vi "load.vi"(8 "error in (no error)":errorcluster, 10 "child node in":refnum<k20>, 11 "TTL_input in":refnum<class "TTL_input.lvclass">) -> (0 "error out":errorcluster, 2 "child node out":refnum<k20>, 3 "TTL_input out":refnum<class "TTL_input.lvclass">)   [LabVIEW 2013, in "TTL_input.lvclass"]
uses:
  TTL_input.lvclass
  TTL_input.lvclass/TTL_input.ctl
  Globals.vi
  <vilib>/xml/Close Reference(Node).vi
  <resource>/objmgr/DOMUserDefRef.rc
  <vilib>/xml/NI_XML.lvlib
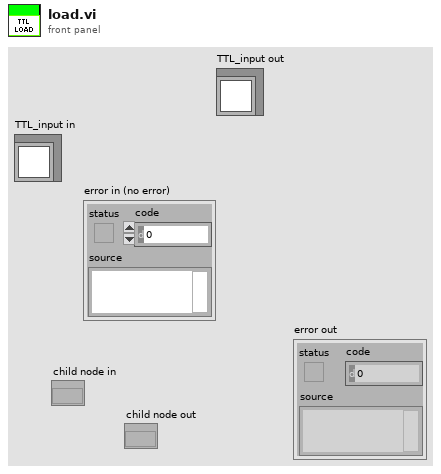
[diagram p1: front panel]
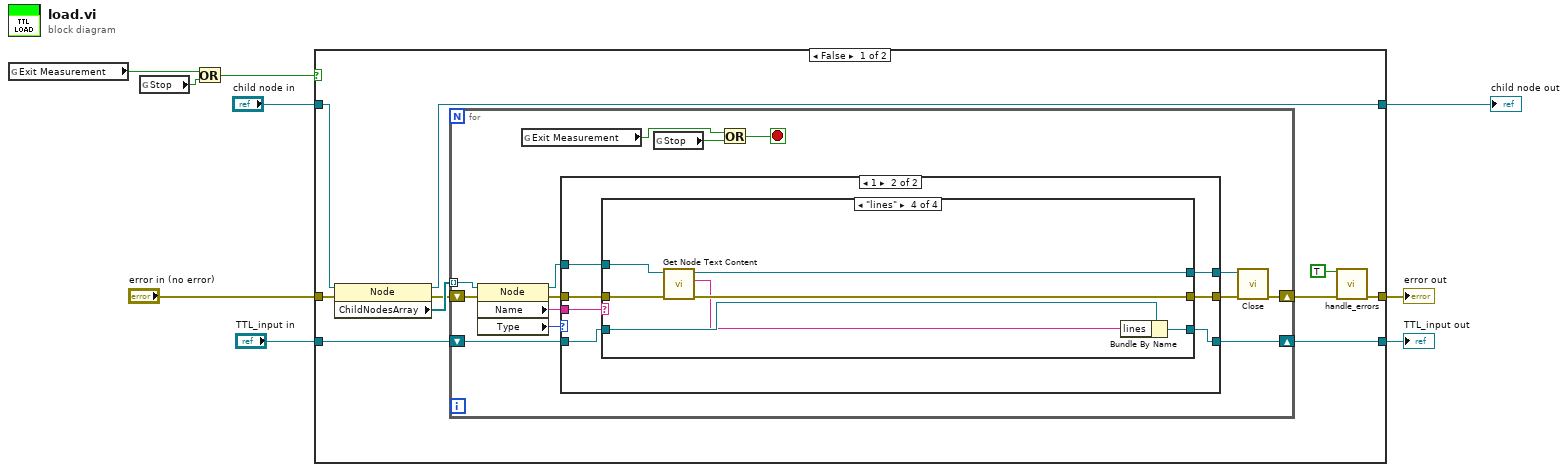
[diagram p0: block diagram]
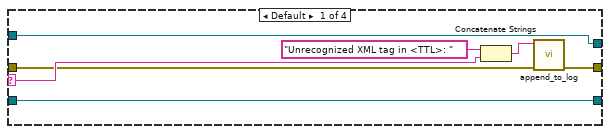
[diagram p3: hidden frame]
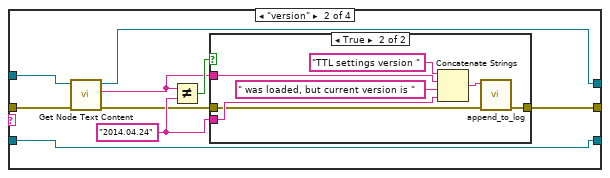
[diagram p4: hidden frame]
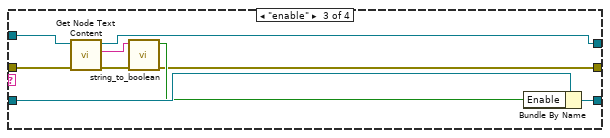
[diagram p6: hidden frame]
diagram:
  n1 = global read "Globals.vi" "Exit Measurement"() -> (w9:bool)
  n2 = global read "Globals.vi" "Stop"() -> (w8:bool)
  n3 = Or(x=w9, y=w8) -> (x .or. y?=w7:bool)
  n4 = case shown="False" w7 {
    tunnel: [w18 w86] -> w3
    tunnel: "error in (no error)" -> [w19 w86]
    tunnel: "TTL_input in" -> [w13 w85]
    tunnel: [w12 w85] -> w4
    tunnel: "child node in" -> [w11 w84]
    tunnel: [w10 w84] -> w1
    frame False {
      n5 = property class="Node"(reference=w11, error in=w19) -> (reference out=w10:refnum<k20>, error out=w16:errorcluster, "ChildNodesArray"=w17:refnum<k20>[])
      n6 = for {
        tunnel: w17 -> [w24] mode=indexing
        shift-right: [w30] -> w12
        shift-left: w13 -> [w31]
        shift-right: [w27] -> w15
        shift-left: w16 -> [w25]
        stop <- w20 stop-if-true
        n7 = property class="Node"(reference=w24, error in=w25) -> (reference out=w32:refnum<k20>, error out=w28:errorcluster, "Name"=w33:string, "Type"=w23:i32)
        n8 = global read "Globals.vi" "Exit Measurement"() -> (w22:bool)
        n9 = case shown="1" w23 {
          tunnel: w33 -> [_ w43]
          tunnel: w32 -> [w36 w42]
          tunnel: w31 -> [w34 w41]
          tunnel: [w34 w40] -> w30
          tunnel: [w36 w39] -> w29
          tunnel: w28 -> [w35 w38]
          tunnel: [w35 w37] -> w26
          frame Default {
          }
          frame 1 {
            n10 = case shown="\"lines\"" w43 {
              selector: w43 -> [w46 _ _ _]
              tunnel: w42 -> [w49 w54 w75 w80]
              tunnel: w41 -> [w50 w53 w73 w83]
              tunnel: [w50 w53 w72 w82] -> w40
              tunnel: [w49 w52 w76 w81] -> w39
              tunnel: w38 -> [w45 w55 w74 w79]
              tunnel: [w44 w51 w68 w78] -> w37
              frame Default {
                n11 = Concatenate Strings("Unrecognized XML tag in <TTL>: " ("string"), w46) -> (w47:string)
                n12 = call "append_to_log.vi"("error in"=w45, "string"=w47) -> ("error out"=w44:errorcluster)  [unwired: 9 in]
              }
              frame "version" {
                w57 = "2014.04.24" ("y")
                n13 = call <vilib>:"Get Node Text Content.vi"("error in (no error)"=w55, "node in"=w54) -> ("error out"=w56:errorcluster, "node text"=w58:string, "node out"=w52:refnum<k20>)  [unwired: 7 in]
                n14 = Not Equal?(x=w58, y=w57) -> (x != y?=w59:bool)
                n15 = case shown="True" w59 {
                  tunnel: w58 -> [_ w66]
                  tunnel: w57 -> [_ w64]
                  tunnel: w56 -> [w60 w62]
                  tunnel: [w60 w61] -> w51
                  frame False {
                  }
                  frame True {
                    n16 = Concatenate Strings("TTL settings version " ("string"), w66, " was loaded, but current version is " ("string"), w64) -> (w63:string)
                    n17 = call "append_to_log.vi"("error in"=w62, "string"=w63) -> ("error out"=w61:errorcluster)  [unwired: 9 in]
                  }
                }
              }
              frame "enable" {
                n18 = call <vilib>:"Get Node Text Content.vi"("error in (no error)"=w74, "node in"=w75) -> ("error out"=w70:errorcluster, "node text"=w71:string, "node out"=w76:refnum<k20>)  [unwired: 7 in]
                n19 = call "string_to_boolean.vi"("error in"=w70, "string"=w71) -> ("error out"=w68:errorcluster, "boolean"=w69:bool)  [unwired: 8 in]
                n20 = Bundle By Name(cluster=w73, "Enable"=w69) -> (w72:refnum<class "TTL_input.lvclass">)
              }
              frame "lines" {
                n21 = call <vilib>:"Get Node Text Content.vi"("error in (no error)"=w79, "node in"=w80) -> ("error out"=w78:errorcluster, "node text"=w77:string, "node out"=w81:refnum<k20>)  [unwired: 7 in]
                n22 = Bundle By Name(cluster=w83, "lines"=w77) -> (w82:refnum<class "TTL_input.lvclass">)
              }
            }
          }
        }
        n23 = global read "Globals.vi" "Stop"() -> (w21:bool)
        n24 = Or(x=w22, y=w21) -> (x .or. y?=w20:bool)
        n25 = call-poly <vilib>:"Close.vi"("error in (no error)"=w26, "node"=w29) -> ("error out"=w27:errorcluster)  [unwired: 7 in]
      }
      n26 = call "handle_errors.vi"("Exit Operation"=TRUE, "error in (no error)"=w15) -> ("error out"=w18:errorcluster)  [unwired: 13 in]
    }
    frame True {
    }
  }
  "error out" <- w3
  "TTL_input out" <- w4
  "child node out" <- w1
